vi "MT Rician Fading Profile (Gans).vi"(0 "profile length (samples)":i32=1000, 1 "rician parameter K (dB)":dbl format="%.2f", 5 "sampling frequency (Hz)":dbl=1.0 format="%.2f", 7 "doppler spread (Hz)":dbl=0.01 format="%.2p", 9 "seed in (0xFFFFFFFF)":i32=-1 format="%.0x", 11 "error in (no error)":errorcluster, 12 "fading variance":dbl=1.0 format="%.2f", 13 "reset? (T)":bool=TRUE) -> (4 "fading profile":cdb[](array[numeric]) format="%.2f", 10 "seed out":i32 format="%.0x", 15 "error out":errorcluster)   [LabVIEW 2020, in "niDMT.lvlib"]
doc: "This polymorphic instance generates a Rician flat-fading profile for the multipath channel. The envelope for the first path statistically obeys the Rician distribution, while the envelope for the remaining path obeys the Rayleigh distribution implemented using the Gans model."
uses:
  <vilib>/addons/Modulation/niDMT.lvlib
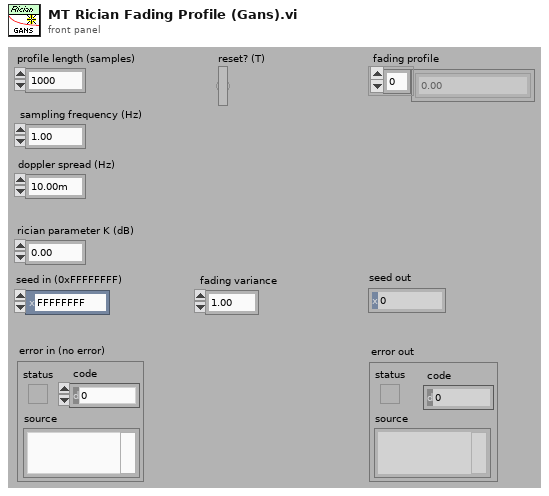
[diagram p1: front panel]
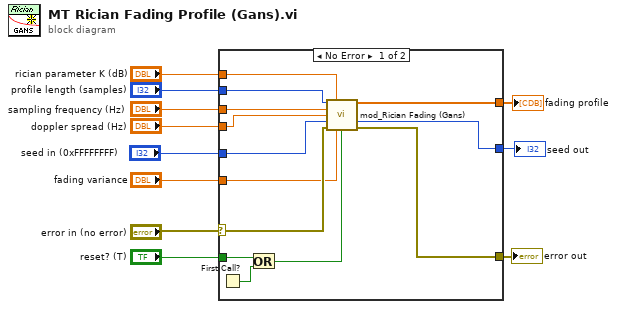
[diagram p0: block diagram]
diagram:
  n1 = case shown="No Error" "error in (no error)" {
    selector: "error in (no error)" -> [w19 w25]
    tunnel: "profile length (samples)" -> [w22 _]
    tunnel: [w24 _] -> w10
    tunnel: [w23 w25] -> w9
    tunnel: "sampling frequency (Hz)" -> [w21 _]
    tunnel: "doppler spread (Hz)" -> [w20 _]
    tunnel: "reset? (T)" -> [w18 _]
    tunnel: "seed in (0xFFFFFFFF)" -> [w15 _]
    tunnel: "rician parameter K (dB)" -> [w14 _]
    tunnel: "fading variance" -> [w13 _]
    tunnel: [w12 _] -> w1
    frame No Error {
      n2 = First Call?() -> (First Call?: T/F=w17:bool)
      n3 = Or(x=w18, y=w17) -> (x .or. y?=w16:bool)
      n4 = call <vilib>:"mod_Rician Fading (Gans).vi"("profile length (samples)"=w22, "rician parameter K (dB)"=w14, "sampling frequency (Hz)"=w21, "doppler spread (Hz)"=w20, "seed in (0xFFFFFFFF)"=w15, "error in (no error)"=w19, "fading variance"=w13, "reset? (T)"=w16) -> ("rician fading profile"=w24:cdb[], "next seed"=w12:i32, "error out"=w23:errorcluster)  [unwired: 5 out]
    }
    frame Error {
    }
  }
  "fading profile" <- w10
  "error out" <- w9
  "seed out" <- w1
